vi "Get Plot Data.vi"(6 "Index":i32, 7 "3D Plot Datatype.lvclass in":refnum<class "3D Plot Datatype.lvclass">, 8 "error in (no error)":errorcluster, 10 "Plot Representation In":T1, 11 "3D Plot.lvclass in":refnum<class "3D Plot.lvclass">) -> (0 "error out":errorcluster, 2 "Plot Representation Out":T1, 3 "3D Plot.lvclass out":refnum<class "3D Plot.lvclass">, 5 "3D Plot Datatype.lvclass out":refnum<class "3D Plot Datatype.lvclass">)   [LabVIEW 2020, in "3D Plot Datatype.lvclass"]
uses:
  3D Plot Datatype.lvclass
  Multiplot Representation.ctl
  Plot Representation.ctl
  Range Clusters.ctl
  Mesh Data.ctl
  3D Plot.lvclass
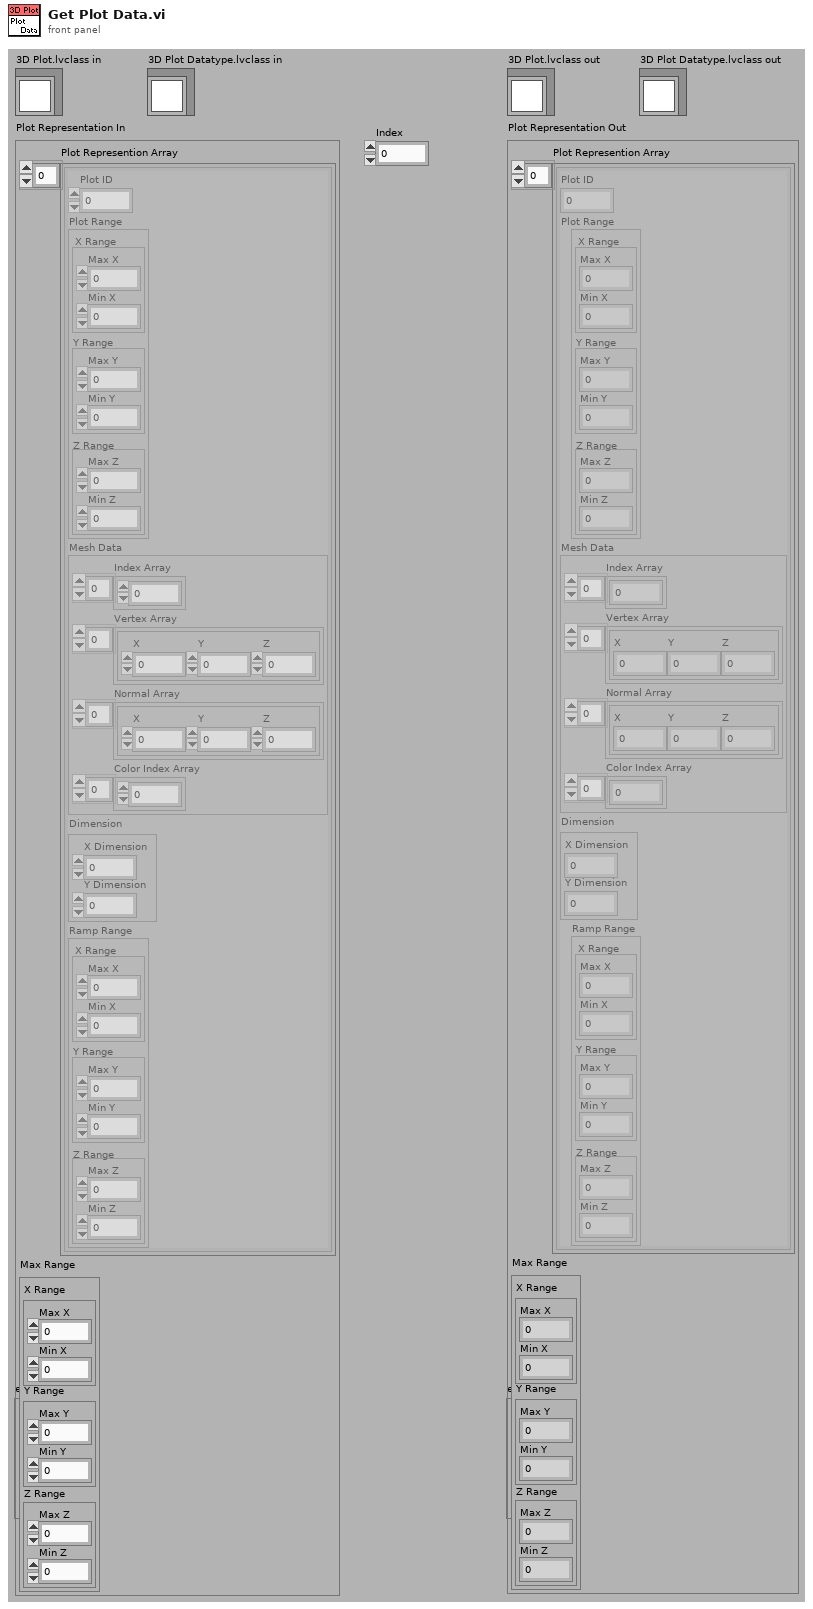
[diagram p1: front panel]
types:
  T1 = typedef "3D Plot.lvclass/Multiplot Representation.ctl" = cluster{"Plot Represention Array":T2[], "Max Range":T3}
  T2 = typedef "3D Plot.lvclass/Plot Representation.ctl" = cluster{"Plot ID":i32, "Plot Range":T3, "Mesh Data":T4, "Dimension":cluster{"X Dimension":i32, "Y Dimension":i32}, "Ramp Range":T3}
  T3 = typedef "3D Plot.lvclass/Range Clusters.ctl" = cluster{"X Range":cluster{"Max X":sgl, "Min X":sgl}, "Y Range":cluster{"Max Y":sgl, "Min Y":sgl}, "Z Range":cluster{"Max Z":sgl, "Min Z":sgl}}
  T4 = typedef "3D Plot.lvclass/Mesh Data.ctl" = cluster{"Index Array":u32[], "Vertex Array":cluster{"X":sgl, "Y":sgl, "Z":sgl}[], "Normal Array":cluster{"X":sgl, "Y":sgl, "Z":sgl}[], "Color Index Array":i32[]}
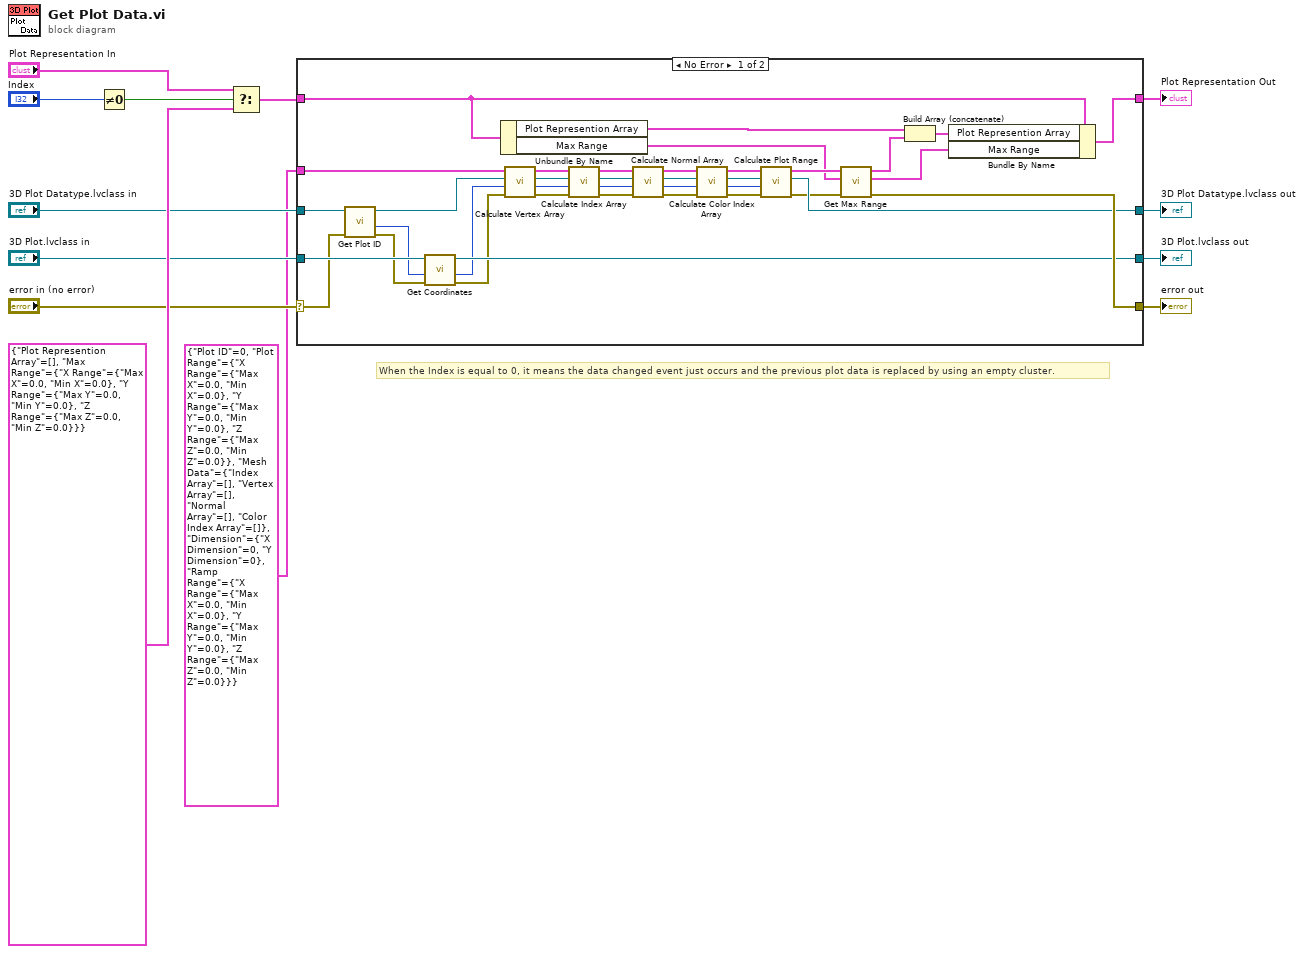
[diagram p0: block diagram]
diagram:
  # "When the Index is equal to 0, it means the data changed event just occurs and the previous plot data is replaced by using an empty cluster."
  n1 = Not Equal To 0?(x="Index") -> (x != 0?=w13:bool)
  n2 = Select(t="Plot Representation In", s=w13, f=T1 {"Plot Represention Array"=[], "Max Range"={"X Range"={"Max X"=0.0, "Min X"=0.0}, "Y Range"={"Max Y"=0.0, "Min Y"=0.0}, "Z Range"={"Max Z"=0.0, "Min Z"=0.0}}}) -> (s? t:f=w9:T1)
  n3 = case shown="No Error" "error in (no error)" {
    selector: "error in (no error)" -> [w29 w52]
    tunnel: [w41 w52] -> w5
    tunnel: w9 -> [w43 w51]
    tunnel: [w42 w51] -> w6
    tunnel: "3D Plot Datatype.lvclass in" -> [w31 w50]
    tunnel: [w37 w50] -> w7
    tunnel: [w34 w49] -> w4
    tunnel: "3D Plot.lvclass in" -> [w35 w49]
    tunnel: T2 {"Plot ID"=0, "Plot Range"={"X Range"={"Max X"=0.0, "Min X"=0.0}, "Y Range"={"Max Y"=0.0, "Min Y"=0.0}, "Z Range"={"Max Z"=0.0, "Min Z"=0.0}}, "Mesh Data"={"Index Array"=[], "Vertex Array"=[], "Normal Array"=[], "Color Index Array"=[]}, "Dimension"={"X Dimension"=0, "Y Dimension"=0}, "Ramp Range"={"X Range"={"Max X"=0.0, "Min X"=0.0}, "Y Range"={"Max Y"=0.0, "Min Y"=0.0}, "Z Range"={"Max Z"=0.0, "Min Z"=0.0}}} ("Plot Representation In") -> [w14 _]
    frame No Error {
      n4 = call-dynamic "Get Plot ID.vi"("error in (no error)"=w29, "3D Plot Datatype.lvclass in"=w31) -> ("error out"=w28:errorcluster, "Plot ID"=w32:i32, "3D Plot Datatype.lvclass out"=w30:refnum<class "3D Plot Datatype.lvclass">)  [unwired: 7 out]
      n5 = call-dynamic "Get Coordinates.vi"("error in (no error)"=w28, "Plot ID"=w32, "3D Plot.lvclass in"=w35) -> ("error out"=w33:errorcluster, "Coordinates System"=w23:enum16{"Cartesian", "Cylindrical", "Spherical"}, "3D Plot.lvclass out"=w34:refnum<class "3D Plot.lvclass">)  [unwired: 6 out]
      n6 = Unbundle By Name(w43) -> ("Plot Represention Array"=w44:T2[], "Max Range"=w26:T3)
      n7 = call-dynamic "Calculate Vertex Array.vi"("error in (no error)"=w33, "Coordinates System"=w23, "3D Plot Datatype.lvclass in"=w30, "Plot Representation In"=w14) -> ("error out"=w46:errorcluster, "Dup Coordinates System"=w16:enum16{"Cartesian", "Cylindrical", "Spherical"}, "3D Plot Datatype.lvclass out"=w40:refnum<class "3D Plot Datatype.lvclass">, "Plot Representation Out"=w48:T2)  [unwired: 4 out]
      n8 = call-dynamic "Calculate Index Array.vi"("error in (no error)"=w46, "3D Plot Datatype.lvclass in"=w40, "Plot Representation In"=w48) -> ("error out"=w45:errorcluster, "3D Plot Datatype.lvclass out"=w39:refnum<class "3D Plot Datatype.lvclass">, "Plot Representation Out"=w47:T2)  [unwired: 6 out]
      n9 = call-dynamic "Calculate Normal Array.vi"("error in (no error)"=w45, "Coordinates System"=w16, "3D Plot Datatype.lvclass in"=w39, "Plot Representation In"=w47) -> ("error out"=w20:errorcluster, "Dup Coordinates System"=w15:enum16{"Cartesian", "Cylindrical", "Spherical"}, "3D Plot Datatype.lvclass out"=w21:refnum<class "3D Plot Datatype.lvclass">, "Plot Representation Out"=w22:T2)  [unwired: 4 out]
      n10 = call-dynamic "Calculate Color Index Array.vi"("error in (no error)"=w20, "3D Plot Datatype in"=w21, "Plot Representation In"=w22) -> ("error out"=w17:errorcluster, "3D Plot Datatype out"=w18:refnum<class "3D Plot Datatype.lvclass">, "Plot Representation Out"=w19:T2)  [unwired: 1 in, 5 out]
      n11 = call-dynamic "Calculate Plot Range.vi"("error in (no error)"=w17, "Coordinates System"=w15, "3D Plot Datatype.lvclass in"=w18, "Plot Representation In"=w19) -> ("error out"=w36:errorcluster, "3D Plot Datatype.lvclass out"=w37:refnum<class "3D Plot Datatype.lvclass">, "Plot Representation Out"=w27:T2)  [unwired: 5 out]
      n12 = call "Get Max Range.vi"("error in (no error)"=w36, "Max Range In"=w26, "Plot Representation In"=w27) -> ("error out"=w41:errorcluster, "Max Range Out"=w24:T3, "Plot Representation Out"=w25:T2)  [unwired: 6 out]
      n13 = Build Array (concatenate)(w44, w25) -> (w38:T2[])
      n14 = Bundle By Name(cluster=w43, "Plot Represention Array"=w38, "Max Range"=w24) -> (w42:T1)
    }
    frame Error {
    }
  }
  "error out" <- w5
  "Plot Representation Out" <- w6
  "3D Plot Datatype.lvclass out" <- w7
  "3D Plot.lvclass out" <- w4
